vi "Pascalstriangle.vi"(11 "dimension size":i32) -> (3 "Array":dbl[](array[numeric]))   [LabVIEW 2015]
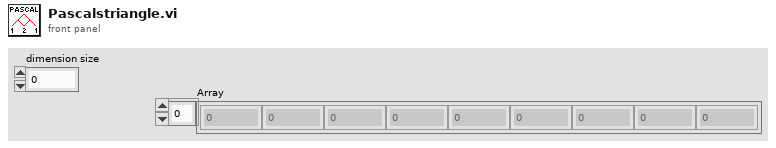
[diagram p1: front panel]
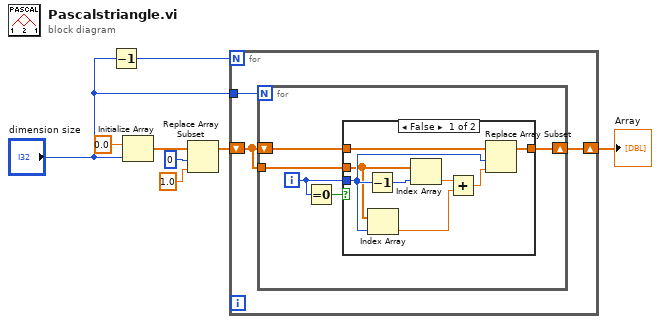
[diagram p0: block diagram]
diagram:
  n1 = Decrement(x="dimension size") -> (x-1=w1:i32)
  n2 = Initialize Array(0.0 ("element"), "dimension size") -> (w7:dbl[])
  n3 = Replace Array Subset(array=w7, new element=1.0 ("new element/subarray"), index=0) -> (w4:dbl[])
  n4 = for {
    N: w1 -> [_]
    tunnel: "dimension size" -> [w11]
    shift-right: [w9] -> w3
    shift-left: w4 -> [w10]
    n5 = for {
      N: w11 -> [_]
      shift-right: [w14] -> w9
      shift-left: w10 -> [w16]
      tunnel: w10 -> [w12]
      i -> [w13]
      n6 = Equal To 0?(x=w13) -> (x = 0?=w15:bool)
      n7 = case shown="False" w15 {
        tunnel: w16 -> [w17 w25]
        tunnel: [w19 w25] -> w14
        tunnel: w13 -> [w21 _]
        tunnel: w12 -> [w18 _]
        frame False {
          n8 = Decrement(x=w21) -> (x-1=w24:i32)
          n9 = Index Array(array=w18, index=w21) -> (element=w22:dbl)
          n10 = Index Array(array=w18, index=w24) -> (element=w23:dbl)
          n11 = Add(x=w23, y=w22) -> (x+y=w20:dbl)
          n12 = Replace Array Subset(array=w17, new element=w20, index=w21) -> (w19:dbl[])
        }
        frame True {
        }
      }
    }
  }
  "Array" <- w3
